vi "Write Enable Bias.vi"(10 "Enable Bias":bool, 11 "LCR-Measurement in":refnum<class "LCR-Meas.lvclass">) -> (3 "LCR-Measurement out":refnum<class "LCR-Meas.lvclass">)   [LabVIEW 2020, in "LCR-Meas.lvclass"]
uses:
  LCR-Meas.lvclass
  LCR-Meas.lvclass/LCR-Meas.ctl
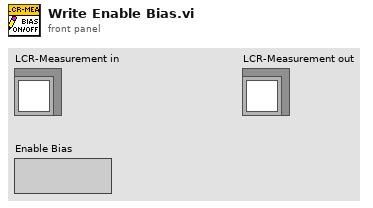
[diagram p1: front panel]
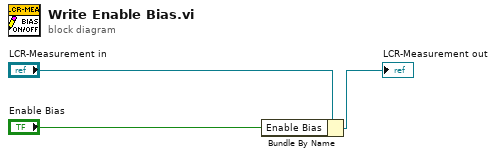
[diagram p0: block diagram]
diagram:
  n1 = Bundle By Name(cluster="LCR-Measurement in", "Enable Bias"="Enable Bias") -> (→"LCR-Measurement out":refnum<class "LCR-Meas.lvclass">)
